vi "Configure Frequency (Start Stop).vi"(0 "VISA resource name":refnum<visa-resource-name>, 7 "Start Frequency (9E+3 Hz)":dbl=9000.0, 11 "error in (no error)":errorcluster, 12 "Stop Frequency (7E+9 Hz)":dbl=7000000000.0) -> (4 "VISA resource name out":refnum<visa-resource-name>, 15 "error out":errorcluster)   [LabVIEW 2022 SP3, in "Agilent N934X Series.lvlib"]
doc: "Configures the frequency range defining its start frequency and its stop frequency. If the start frequency is equal to the stop frequency, then the spectrum analyzer operates in the time-domain mode. Otherwise, the spectrum analyzer operates in frequency-domain mode."
uses:
  <instrlib>/Agilent N934X Series/Agilent N934X Series.lvlib
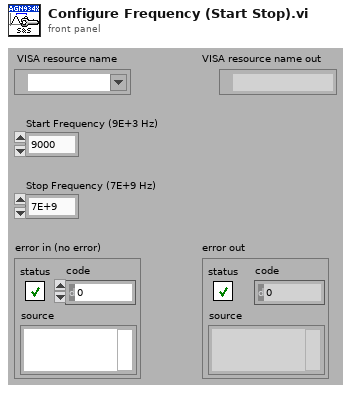
[diagram p1: front panel]
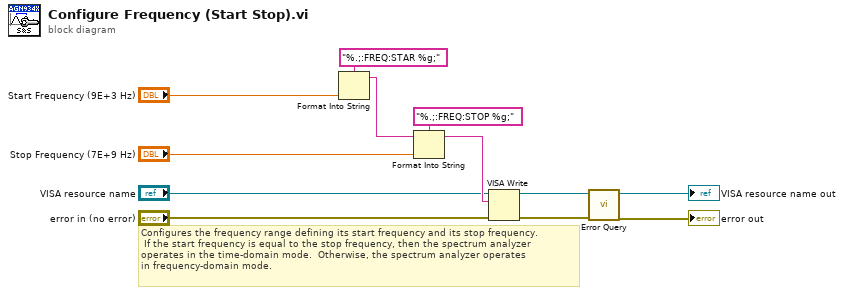
[diagram p0: block diagram]
diagram:
  # "Configures the frequency range defining its start frequency and its stop frequency. \n If the start frequency is equal to the stop frequency, then the spectrum analyzer \noperates in the time-domain mode.  Otherwise, the spectrum analyzer operates \nin frequency-domain mode."
  n1 = Format Into String(format string="%.;:FREQ:STAR %g;", "Start Frequency (9E+3 Hz)") -> (resulting string=w10:string)  [unwired: 2 in, 1 out]
  n2 = Format Into String(format string="%.;:FREQ:STOP %g;", initial string=w10, "Stop Frequency (7E+9 Hz)") -> (resulting string=w7:string)  [unwired: 1 in, 1 out]
  n3 = VISA Write(VISA resource name="VISA resource name", write buffer=w7, error in (no error)="error in (no error)") -> (VISA resource name out=w4:refnum<visa-resource-name>, error out=w3:errorcluster)  [unwired: 1 out]
  n4 = call <instrlib>:"Error Query.vi"("error in (no error)"=w3, "VISA resource name"=w4) -> ("error out"=→"error out":errorcluster, "VISA resource name out"=→"VISA resource name out":refnum<visa-resource-name>)  [unwired: 6 in, 2 out]
